vi "DCM Constants and GUIDs.vi"() -> ()   [LabVIEW 2016, in "DCM Shared.lvlib"]
uses:
  DCM Shared.lvlib
  Types/Channel.ctl
panel:
  in  "Tab Control":T1(tab)
  in  "GUID.Aux":string="4ae80cd4-ec55-4ec1-b4bb-2001c61b6b14"
  in  "GUID.EnableDisableKnock":string="8a875cae-6cab-46b6-b4a7-b8cdf862ac1d"
  in  "GUID.Knock Disabled":string="a0532e73-7f55-4d0e-9b0f-dca8ef6be3da"
  in  "GUID.EnableDisableSkipfire":string="bbdda3d2-34c9-4362-989f-a288134847eb"
  in  "GUID.Skipfire Disabled":string="c54507d4-3cef-40f9-a6c1-87c28a1ea6a0"
  in  "GUID.Skipfire":string="1ac39163-a8a7-406d-af0d-2094f9d35b5e"
  in  "GUID.HH Scope":string="6092b7fa-6603-4513-a21d-943bed09a899"
  in  "GUID.EnableDisableESTTL":string="e242de91-e1a9-42ca-a209-c7115f438d37"
  in  "GUID.ESTTL Disabled":string="2ad3d1d5-7c00-47db-b770-0db9f08c91b8"
  in  "GUID.EnableDisableDiffIO":string="917ddf8a-c153-44a1-b2f2-6ada7a308212"
  in  "GUID.Differential IO Disabled":string="faee9789-46db-458a-959a-05641d5004e2"
  in  "GUID.EnableDisableHalfH":string="e0f39d5d-4753-4142-ac63-84ba8dc69499"
  in  "GUID.Half-H Disabled":string="e47a1de0-27ee-4cc7-82d3-285b476618bb"
  in  "GUID.EnableDisableBankB":string="4d434972-4aa6-45af-92be-8034ae6f2b6c"
  in  "GUID.EnableDisableBankA":string="46df0418-deb6-4d59-8d20-0ae52d1e3a0a"
  in  "GUID.DI (Bank B) Disabled":string="ba7b8b99-1cfb-447e-88fa-e4ec3244df79"
  in  "GUID.DI (Bank A) Disabled":string="0515dfd1-3106-4f60-bfdc-e9560b274cce"
  in  "GUID.Knock":string="19fe4c45-3921-4e09-b642-633bf2891a16"
  in  "GUID.UEGO":string="5fb3e6f2-894a-4878-a5bb-3886d90bfc3e"
  in  "GUID.VR-Hall":string="cf54691f-9754-47a4-ae55-d66845591b75"
  in  "GUID.ESTTL":string="38e1f48f-5a27-4a02-97fd-d113d0b0a1a5"
  in  "GUID.Wvfrm Del Prot":string="7d419a3c-75c3-4347-a0a2-a7591295b469"
  in  "GUID.System":string="d2cc065c-850f-4944-a4c9-610c3de05f2d"
  in  "GUID.Sect Write Del Prot":string="e1e0ebe0-7744-485e-8dcf-da45db37f6d7"
  in  "GUID.DI Scope":string="4a79ddeb-a706-489a-9bbf-290de6baccd6"
  in  "GUID.EnableDisableMain":string="f10bd84a-c71b-4bab-a7fa-9098b9fd69a6"
  in  "GUID.Status":string="39854a26-935c-4763-8ef8-825ef45b52f8"
  in  "GUID.Main Disabled":string="f599dfb9-ed26-42aa-8cdc-f57f090e1b11"
  in  "GUID.Differential IO":string="2628923f-4c3d-4e64-9018-fe4e0bf24e80"
  in  "GUID.Half-H":string="f16175a1-fad9-427d-a4ec-263940a8031d"
  in  "GUID.DI (Bank B)":string="a63b3095-c73b-454f-88f9-68383dab1f80"
  in  "GUID.DI (Bank A)":string="f8d973f8-2e11-4124-aa70-a6fee72385c1"
  in  "GUID.EPTx":string="a5efee57-fd86-4078-b618-b0705acc47b3"
  in  "GUID.Sect Read Del Prot":string="6b94385d-a8fe-4299-8780-02040b069697"
  in  "GUID.Chan Del Prot":string="c457cef7-60a4-4609-953f-49bd172293ff"
  in  "GUID.Main Enabled":string="1e4c05d8-9abf-4fec-b650-9db71821173c"
  in  "Constant.Aux Inputs":string="Aux Inputs"
  in  "Constant.Skip Fire":string="Skip Fire"
  in  "Constant.Select 2":string="Select"
  in  "Constant.Filters":string="Filters"
  in  "Constant.Half-H Scope":string="Half-H Scope"
  in  "Constant.Command DI":string="Command DI"
  in  "Constant.Command Pump":string="Command Pump"
  in  "Constant.Knock Intensity":string="Knock Intensity"
  in  "Constant.Knock":string="Knock"
  in  "Constant.Diagnostics":string="Diagnostics"
  in  "Constant.Temperature":string="Temperature"
  in  "Constant.ESTTL":string="ESTTL"
  in  "Constant.VR-Hall":string="VR-Hall"
  in  "Constant.UEGO":string="UEGO"
  in  "Constant.Invalid Selection":string="Invalid Selection"
  in  "Constant.WrongMode":string="Selected Configuration invalid for Sync Pump operation."
  in  "Constant.Select":string="Select"
  in  "Constant.User OS":string="User OS"
  in  "Constant.Config":string="Config"
  in  "Constant.DisableChannels":string="Disabling channels will delete all relevant configuration information. Proceed?"
  in  "Constant.Input State":string="Input State"
  in  "Constant.Clear Faults":string="Clear Faults"
  in  "Constant.Debug":string="Debug"
  in  "Constant.Mux ADC":string="Mux ADC"
  in  "Constant.System":string="System"
  in  "Constant.DI Scope":string="DI Scope"
  in  "Constant.Description":string="Description"
  in  "Constant.HH Command":string="HH Command"
  in  "Constant.Results":string="Results"
  in  "Constant.Setup":string="Setup"
  in  "Constant.Command":string="Command"
  in  "Constant.EPTx":string="EPTx"
  in  "Constant.invalid bitfile":string="Invalid Bitfile"
  in  "Constant.ConfirmDelete":string="Confirm delete configuration"
  in  "Constant.ChangeBitfile":string="Changing bitfile will delete all relevant configuration information. Proceed?"
  in  "Constant.RemoveBitfile":string="Removing the bitfile path will delete all configuration information. Proceed?"
  in  "Constant.Status":string="Status"
  in  "Constant.Waveforms":string="Waveforms"
  in  "Constant.Thresholding":string="Thresholding"
  in  "Constant.Differential IO":string="Differential I/O"
  in  "Constant.Half-H":string="Half-H"
  in  "Constant.DI (Bank B)":string="DI (Bank B)"
  in  "Constant.DI (Bank A)":string="DI (Bank A)"
  in  "Constant.Data":string="Data"
  in  "Constant.Control":string="Control"
  in  "Constant.not present":string="- not added -"
  in  "ChanList.DI Status":T2[](array[typedef])=[{"Name"="A Run State", "Units"="enum", "Default"=0.0, "Description"="Indicates DI Bank A run status. [Idle|Warmup|Ready to Inject|Cooldown]"}, {"Name"="B Run State", "Units"="enum", "Default"=0.0, "Description"="Indicates DI Bank B run status. [Idle|Warmup|Ready to Inject|Cooldown]"}]
  in  "ChanList.Knock Controls":T2[](array[typedef])=[{"Name"="Low Cutoff", "Units"="Hz", "Default"=4000.0, "Description"="Sets the low cutoff frequency for knock calculations."}, {"Name"="High Cutoff", "Units"="Hz", "Default"=10000.0, "Description"="Sets the high cutoff frequency for knock calculations."}, {"Name"="Threshold", "Units"="", "Default"=1.0, "Description"="Sets the minimum calculation result which represents a knocking condition."}, {"Name"="Knock Start", "Units"="CAD", "Default"=0.0, "Description"="Sets the start of the knock sampling window."}, {"Name"="Knock End", "Units"="CAD", "Default"=0.0, "Description"="Sets the end of the knock sampling window."}, {"Name"="Reference Start", "Units"="CAD", "Default"=0.0, "Description"="Sets the start of the reference sampling window."}, {"Name"="Reference End", "Units"="CAD", "Default"=0.0, "Description"="Sets the end of the reference sampling window."}]
  in  "ChanList.HH Scope":T2[](array[typedef])=[{"Name"="Capture Enable", "Units"="bool", "Default"=0.0, "Description"="Enables HH-ADC Scope capture."}, {"Name"="Capture Event", "Units"="enum", "Default"=0.0, "Description"="Selects the HH-ADC scope trigger event."}, {"Name"="Capture Length", "Units"="s", "Default"=0.0, "Description"="Sets the length of the HH Scope waveform buffer."}, {"Name"="dt", "Units"="s", "Default"=2e-07, "Description"="Indicates the HH Scope dt in seconds."}]
  in  "ChanList.Knock Intensity":T2[](array[typedef])=[{"Name"="Knock Intensity 1", "Units"="", "Default"=0.0, "Description"="Indicates the intensity of knock reported by the FPGA."}, {"Name"="Knock Intensity 2", "Units"="", "Default"=0.0, "Description"="Indicates the intensity of knock reported by the FPGA."}, {"Name"="Knock Intensity 3", "Units"="", "Default"=0.0, "Description"="Indicates the intensity of knock reported by the FPGA."}, {"Name"="Knock Intensity 4", "Units"="", "Default"=0.0, "Description"="Indicates the intensity of knock reported by the FPGA."}, {"Name"="Knock Intensity 5", "Units"="", "Default"=0.0, "Description"="Indicates the intensity of knock reported by the FPGA."}, {"Name"="Knock Intensity 6", "Units"="", "Default"=0.0, "Description"="Indicates the intensity of knock reported by the FPGA."}, {"Name"="Knock Intensity 7", "Units"="", "Default"=0.0, "Description"="Indicates the intensity of knock reported by the FPGA."}, {"Name"="Knock Intensity 8", "Units"="", "Default"=0.0, "Description"="Indicates the intensity of knock reported by the FPGA."}, {"Name"="Knock Intensity 9", "Units"="", "Default"=0.0, "Description"="Indicates the intensity of knock reported by the FPGA."}, {"Name"="Knock Intensity 10", "Units"="", "Default"=0.0, "Description"="Indicates the intensity of knock reported by the FPGA."}, {"Name"="Knock Intensity 11", "Units"="", "Default"=0.0, "Description"="Indicates the intensity of knock reported by the FPGA."}, {"Name"="Knock Intensity 12", "Units"="", "Default"=0.0, "Description"="Indicates the intensity of knock reported by the FPGA."}, {"Name"="Knock Intensity 13", "Units"="", "Default"=0.0, "Description"="Indicates the intensity of knock reported by the FPGA."}, {"Name"="Knock Intensity 14", "Units"="", "Default"=0.0, "Description"="Indicates the intensity of knock reported by the FPGA."}, {"Name"="Knock Intensity 15", "Units"="", "Default"=0.0, "Description"="Indicates the intensity of knock reported by the FPGA."}, {"Name"="Knock Intensity 16", "Units"="", "Default"=0.0, "Description"="Indicates the intensity of knock reported by the FPGA."}]
  in  "ChanList.Knock Result":T2[](array[typedef])=[{"Name"="Knock 1", "Units"="bool", "Default"=0.0, "Description"="Indicates the presence of knock above the calibrated threshold."}, {"Name"="Knock 2", "Units"="bool", "Default"=0.0, "Description"="Indicates the presence of knock above the calibrated threshold."}, {"Name"="Knock 3", "Units"="bool", "Default"=0.0, "Description"="Indicates the presence of knock above the calibrated threshold."}, {"Name"="Knock 4", "Units"="bool", "Default"=0.0, "Description"="Indicates the presence of knock above the calibrated threshold."}, {"Name"="Knock 5", "Units"="bool", "Default"=0.0, "Description"="Indicates the presence of knock above the calibrated threshold."}, {"Name"="Knock 6", "Units"="bool", "Default"=0.0, "Description"="Indicates the presence of knock above the calibrated threshold."}, {"Name"="Knock 7", "Units"="bool", "Default"=0.0, "Description"="Indicates the presence of knock above the calibrated threshold."}, {"Name"="Knock 8", "Units"="bool", "Default"=0.0, "Description"="Indicates the presence of knock above the calibrated threshold."}, {"Name"="Knock 9", "Units"="bool", "Default"=0.0, "Description"="Indicates the presence of knock above the calibrated threshold."}, {"Name"="Knock 10", "Units"="bool", "Default"=0.0, "Description"="Indicates the presence of knock above the calibrated threshold."}, {"Name"="Knock 11", "Units"="bool", "Default"=0.0, "Description"="Indicates the presence of knock above the calibrated threshold."}, {"Name"="Knock 12", "Units"="bool", "Default"=0.0, "Description"="Indicates the presence of knock above the calibrated threshold."}, {"Name"="Knock 13", "Units"="bool", "Default"=0.0, "Description"="Indicates the presence of knock above the calibrated threshold."}, {"Name"="Knock 14", "Units"="bool", "Default"=0.0, "Description"="Indicates the presence of knock above the calibrated threshold."}, {"Name"="Knock 15", "Units"="bool", "Default"=0.0, "Description"="Indicates the presence of knock above the calibrated threshold."}, {"Name"="Knock 16", "Units"="bool", "Default"=0.0, "Description"="Indicates the presence of knock above the calibrated threshold."}]
  in  "ChanList.VR-Hall":T2[](array[typedef])=[{"Name"="Clear Faults", "Units"="bool", "Default"=0.0, "Description"="Clears a fault condition where an input voltage is too negative to safely engage pull-up resistor on the positive(+) side of input channels."}]
  in  "ChanList.UEGO Temp":T2[](array[typedef])=[{"Name"="UEGO1Temp", "Units"="C", "Default"=0.0, "Description"="The controlled temperature, in degrees Celsius, of the wide-band sensor element.\n \nFor LSU 4.2 sensors the temperature setpoint is 750 degrees C.\n \nFor LSU 4.9 sensors the temperature setpoint is 780 degrees C.\n \nThe allowable voltage range for LSU 4.X sensor heater operation is 8.0-16.5V, even though the O2 Sensor Module will operate from 7-32V supply.  If the module supply voltage exceeds 16.5V, the sensor heater will be disabled."}, {"Name"="UEGO2Temp", "Units"="C", "Default"=0.0, "Description"="The controlled temperature, in degrees Celsius, of the wide-band sensor element.\n \nFor LSU 4.2 sensors the temperature setpoint is 750 degrees C.\n \nFor LSU 4.9 sensors the temperature setpoint is 780 degrees C.\n \nThe allowable voltage range for LSU 4.X sensor heater operation is 8.0-16.5V, even though the O2 Sensor Module will operate from 7-32V supply.  If the module supply voltage exceeds 16.5V, the sensor heater will be disabled."}, {"Name"="UEGO1Hot", "Units"="bool", "Default"=0.0, "Description"="Indicates whether the sensor ceramic temperature has reached the target after enabled.  Lambda results are valid when UEGOXHot is TRUE.\n \nFor LSU 4.2 :\nA temperature change of the sensor ceramic gives a deviation of the sensor output signal of approximately 6%/100C.\nTarget ceramic temperature: 750C\nUEGOHot transitions from FALSE to TRUE when the temperature reaches the target temperature for the first time after enabled.\nUEGOHot transitions from TRUE to FALSE when the sensor or module are disabled, or the battery voltage is measured out of range.\n \nFor LSU 4.9 :\nA temperature change of the sensor ceramic gives a deviation of the sensor output signal of approximately 4%/100C.\nTarget ceramic temperature: 780C\nUEGOHot transitions from FALSE to TRUE when the temperature reaches the target temperature for the first time after enabled.\nUEGOHot transitions from TRUE to FALSE when the sensor or module are disabled, or the battery voltage is measured out of range.\n \nThe allowable voltage range for LSU 4.X sensor heater operation is 8.0-16.5V, even though the O2 Sensor Module will operate from 7-32V supply.  If the module supply voltage exceeds 16.5V, the sensor heater will be disabled."}, {"Name"="UEGO2Hot", "Units"="bool", "Default"=0.0, "Description"="Indicates whether the sensor ceramic temperature has reached the target after enabled.  Lambda results are valid when UEGOXHot is TRUE.\n \nFor LSU 4.2 :\nA temperature change of the sensor ceramic gives a deviation of the sensor output signal of approximately 6%/100C.\nTarget ceramic temperature: 750C\nUEGOHot transitions from FALSE to TRUE when the temperature reaches the target temperature for the first time after enabled.\nUEGOHot transitions from TRUE to FALSE when the sensor or module are disabled, or the battery voltage is measured out of range.\n \nFor LSU 4.9 :\nA temperature change of the sensor ceramic gives a deviation of the sensor output signal of approximately 4%/100C.\nTarget ceramic temperature: 780C\nUEGOHot transitions from FALSE to TRUE when the temperature reaches the target temperature for the first time after enabled.\nUEGOHot transitions from TRUE to FALSE when the sensor or module are disabled, or the battery voltage is measured out of range.\n \nThe allowable voltage range for LSU 4.X sensor heater operation is 8.0-16.5V, even though the O2 Sensor Module will operate from 7-32V supply.  If the module supply voltage exceeds 16.5V, the sensor heater will be disabled."}]
  in  "ChanList.UEGO Diagnostics":T2[](array[typedef])=[{"Name"="UEGO1SensorFault", "Units"="enum", "Default"=0.0, "Description"="NO FAULT: No faults exist with the sensor signal wires. \n \nSHORT TO GND OR BATT: A short to ground or battery is present on one of the sensor signal wires."}, {"Name"="UEGO2SensorFault", "Units"="enum", "Default"=0.0, "Description"="NO FAULT: No faults exist with the sensor signal wires. \n \nSHORT TO GND OR BATT: A short to ground or battery is present on one of the sensor signal wires."}, {"Name"="UEGO1HeaterFault", "Units"="enum", "Default"=0.0, "Description"="NO FAULT: No faults exist with the sensor heater wires. \n \nSHORT TO GROUND: A short to ground is present on one of the sensor heater wires. \n \nOPEN CIRCUIT: An open circuit is present on one of the sensor heater wires. \n \nSHORT TO BATTERY: A short to battery is present on one of the sensor heater wires."}, {"Name"="UEGO2HeaterFault", "Units"="enum", "Default"=0.0, "Description"="NO FAULT: No faults exist with the sensor heater wires. \n \nSHORT TO GROUND: A short to ground is present on one of the sensor heater wires. \n \nOPEN CIRCUIT: An open circuit is present on one of the sensor heater wires. \n \nSHORT TO BATTERY: A short to battery is present on one of the sensor heater wires."}, {"Name"="UEGOFuseStatus", "Units"="enum", "Default"=0.0, "Description"="A single fuse is located in the module circuit which feeds battery voltage to both sensor heaters. \n \nFUSE OK: The heater circuit fuse is OK. \n \nFUSE BLOWN: The heater circuit fuse is blown."}, {"Name"="Battery", "Units"="V", "Default"=0.0, "Description"="Battery voltage sensed internal to the module while enabled."}, {"Name"="LSUType", "Units"="enum", "Default"=0.0, "Description"="Indicates the UEGO sensor type supported by the module according to an internal mechanical switch.\n \nFALSE (default switch position): Module switch is configured for the Bosch LSU 4.9 sensor.\n \nTRUE: Module switch is configured for the Bosch LSU 4.2 sensor.\n \nNote: The module can only support one UEGO sensor type.  It is not possible to configure the two UEGO sensor channels for different sensor types.\n \nNote: The NI 9757 module has a single internal mechanical switch that determines the supported sensor type by selecting the correct passive components for the sensors.  This switch is configured from the factory to support the Bosch LSU 4.9 sensor. The UEGO Diagnostics cluster reports the switch configuration.\n \nWARNING: The module does not automatically detect the type of UEGO sensor wired to the module.  If the connected sensor type does not match the module mechanical switch setting, damage may occur to the sensor.  In particular, an LSU 4.9 sensor operated while the switch is set to LSU 4.2 will cause the 4.9 sensor to overheat."}]
  in  "ChanList.UEGO Results":T2[](array[typedef])=[{"Name"="UEGO1Lambda", "Units"="", "Default"=0.0, "Description"="The actual air-fuel mass ratio divided by the stoichiometric air-fuel mass ratio. Lambda is equivalent to 1/Phi."}, {"Name"="UEGO1Phi", "Units"="", "Default"=0.0, "Description"="The actual fuel/air mass ratio divided by the stoichiometric fuel-air mass ratio. Phi is equivalent to 1/Lambda."}, {"Name"="UEGO1AFRatio", "Units"="", "Default"=0.0, "Description"="The actual air-fuel mass ratio."}, {"Name"="UEGO1Ip", "Units"="mA", "Default"=0.0, "Description"="The pump current required for maintaining a reference voltage of 450 millivolts across the wide-band sensor element. This is also the current required for maintaining a stoichiometric gas mixture within the sensor element."}, {"Name"="UEGO2Lambda", "Units"="", "Default"=0.0, "Description"="The actual air-fuel mass ratio divided by the stoichiometric air-fuel mass ratio. Lambda is equivalent to 1/Phi."}, {"Name"="UEGO2Phi", "Units"="", "Default"=0.0, "Description"="The actual fuel/air mass ratio divided by the stoichiometric fuel-air mass ratio. Phi is equivalent to 1/Lambda."}, {"Name"="UEGO2AFRatio", "Units"="", "Default"=0.0, "Description"="The actual air-fuel mass ratio."}, {"Name"="UEGO2Ip", "Units"="mA", "Default"=0.0, "Description"="The pump current required for maintaining a reference voltage of 450 millivolts across the wide-band sensor element. This is also the current required for maintaining a stoichiometric gas mixture within the sensor element."}]
  in  "ChanList.UEGO Control":T2[](array[typedef])=[{"Name"="UEGO1Enable", "Units"="bool", "Default"=0.0, "Description"="Enables UEGO1 sensor"}, {"Name"="UEGO2Enable", "Units"="bool", "Default"=0.0, "Description"="Enables UEGO2 sensor"}, {"Name"="UEGO1Range", "Units"="bool", "Default"=0.0, "Description"="Adjusts the amplifaction range for lambda measurement.  Two amplification modes are available:  One mode, having an amplifier gain factor of 8, allows for measurements of lambda from 0.65 to air.  The other mode, having an amplifier gain factor of 17, allows for measurements of lambda = 0.75 to air.  It is recommended to use the gain factor of 17 for operation above lambda = 1.5.  This gain factor provides better resolution in the lean region.  The gain factor can be changed at any time during operation.\n \nFALSE (Gain factor = 8): Allows measurement of lambda from 0.65 to air.\n \nTRUE (Gain factor = 17): Allows measurement of lambda from 0.75 to air."}, {"Name"="UEGO2Range", "Units"="bool", "Default"=0.0, "Description"="Adjusts the amplifaction range for lambda measurement.  Two amplification modes are available:  One mode, having an amplifier gain factor of 8, allows for measurements of lambda from 0.65 to air.  The other mode, having an amplifier gain factor of 17, allows for measurements of lambda = 0.75 to air.  It is recommended to use the gain factor of 17 for operation above lambda = 1.5.  This gain factor provides better resolution in the lean region.  The gain factor can be changed at any time during operation.\n \nFALSE (Gain factor = 8): Allows measurement of lambda from 0.65 to air.\n \nTRUE (Gain factor = 17): Allows measurement of lambda from 0.75 to air."}, {"Name"="Filter Cutoff", "Units"="Hz", "Default"=10.0, "Description"="Second-order Butterworth lowpass filter cutoff frequency which applies to all UEGO signals."}]
  in  "ChanList.UserOS":T2[](array[typedef])=[{"Name"="User OS", "Units"="bool", "Default"=0.0, "Description"="Triggers a one-shot injection on OS-enabled channels on rising edge."}, {"Name"="User OS Time", "Units"="s", "Default"=0.0, "Description"="One-shot duration in seconds."}]
  in  "ChanList.HH Status":T2[](array[typedef])=[{"Name"="Current", "Units"="A", "Default"=0.0, "Description"="Instantaneous channel current in amps."}, {"Name"="Config Error", "Units"="bool", "Default"=0.0, "Description"="Indicates a configuration error on this channel."}, {"Name"="Short Fault", "Units"="bool", "Default"=0.0, "Description"="Indicates a short is detected on this channel."}, {"Name"="Open Fault", "Units"="bool", "Default"=0.0, "Description"="Indicates an open circuit was detected on this channel."}, {"Name"="Period Min", "Units"="A", "Default"=0.0, "Description"="Min current measured during one command period."}, {"Name"="Period Max", "Units"="A", "Default"=0.0, "Description"="Max current measured during one command period."}, {"Name"="Period Avg", "Units"="A", "Default"=0.0, "Description"="Average current mesasured during one command period"}, {"Name"="On Avg", "Units"="A", "Default"=0.0, "Description"="Average current measured during the on portion of one command period."}]
  in  "ChanList.DiffIO In":T2[](array[typedef])=[{"Name"="DI 1", "Units"="bool", "Default"=0.0, "Description"="Digital state of Diff IO channel input."}, {"Name"="DI 2", "Units"="bool", "Default"=0.0, "Description"="Digital state of Diff IO channel input."}, {"Name"="DI 3", "Units"="bool", "Default"=0.0, "Description"="Digital state of Diff IO channel input."}, {"Name"="DI 4", "Units"="bool", "Default"=0.0, "Description"="Digital state of Diff IO channel input."}, {"Name"="DI 5", "Units"="bool", "Default"=0.0, "Description"="Digital state of Diff IO channel input."}, {"Name"="DI 6", "Units"="bool", "Default"=0.0, "Description"="Digital state of Diff IO channel input."}, {"Name"="DI 7", "Units"="bool", "Default"=0.0, "Description"="Digital state of Diff IO channel input."}, {"Name"="DI 8", "Units"="bool", "Default"=0.0, "Description"="Digital state of Diff IO channel input."}]
  in  "ChanList.DI Fault Clear":T2[](array[typedef])=[{"Name"="Channel 1", "Units"="bool", "Default"=0.0, "Description"="Clears DI faults on this channel."}, {"Name"="Channel 2", "Units"="bool", "Default"=0.0, "Description"="Clears DI faults on this channel."}, {"Name"="Channel 3", "Units"="bool", "Default"=0.0, "Description"="Clears DI faults on this channel."}, {"Name"="Channel 4", "Units"="bool", "Default"=0.0, "Description"="Clears DI faults on this channel."}, {"Name"="Channel 5", "Units"="bool", "Default"=0.0, "Description"="Clears DI faults on this channel."}, {"Name"="Channel 6", "Units"="bool", "Default"=0.0, "Description"="Clears DI faults on this channel."}, {"Name"="Channel 7", "Units"="bool", "Default"=0.0, "Description"="Clears DI faults on this channel."}, {"Name"="Channel 8", "Units"="bool", "Default"=0.0, "Description"="Clears DI faults on this channel."}]
  in  "ChanList.DI Config":T2[](array[typedef])=[{"Name"="Power Supply Enable", "Units"="bool", "Default"=0.0, "Description"="Enables high voltage power supply (0=F, 1=T)."}, {"Name"="Injection Enable", "Units"="bool", "Default"=0.0, "Description"="Enables injection (0=F, 1=T)."}, {"Name"="High Voltage Target", "Units"="V", "Default"=75.0, "Description"="Sets the high voltage power supply target in volts."}]
  in  "ChanList.DI Scope":T2[](array[typedef])=[{"Name"="Capture Enable", "Units"="bool", "Default"=0.0, "Description"="Enables DI-ADC Scope capture."}, {"Name"="Capture Event", "Units"="enum", "Default"=0.0, "Description"="Selects the DI-ADC scope trigger event."}, {"Name"="Capture Length", "Units"="s", "Default"=0.0, "Description"="Sets the length of the DI Scope waveform buffer."}, {"Name"="Channel 1", "Units"="enum", "Default"=0.0, "Description"="Selects the desired channel for the high-speed DI ADC.\n\n0: Lowside Current A1\n1: Lowside Current A2\n2: Lowside Current A3\n3: Lowside Current A4\n4: Lowside Current A5\nA: Piezo Voltage A1\nB: Piezo Voltage A2\nC: Piezo Voltage A3\nD: Piezo Voltage A4\n6: Solenoid Voltage A1\n7: Solenoid Voltage A2\n8: Solenoid Voltage A3\n9: Solenoid Voltage A4\n60: High Voltage A1\n70: High Voltage A2\nE: High Voltage A\n-----------------------------\n13: Lowside Current B1\n12: Lowside Current B2\n11: Lowside Current B3\n10: Lowside Current B4\n14: Lowside Current B5\n19: Piezo Voltage B1\n18: Piezo Voltage B2\n17: Piezo Voltage B3\n16: Piezo Voltage B4\n1F: Solenoid Voltage B1\n1E: Solenoid Voltage B2\n1D: Solenoid Voltage B3\n1C: Solenoid Voltage B4\n90: High Voltage B1\n80: High Voltage B2\nF: High Voltage B\n-----------------------------\n1A: Analog Input 1\n1B: Analog Input 2\nA0: Drive Power"}, {"Name"="Channel 2", "Units"="enum", "Default"=0.0, "Description"="Selects the desired channel for the high-speed DI ADC.\n\n0: Lowside Current A1\n1: Lowside Current A2\n2: Lowside Current A3\n3: Lowside Current A4\n4: Lowside Current A5\nA: Piezo Voltage A1\nB: Piezo Voltage A2\nC: Piezo Voltage A3\nD: Piezo Voltage A4\n6: Solenoid Voltage A1\n7: Solenoid Voltage A2\n8: Solenoid Voltage A3\n9: Solenoid Voltage A4\n60: High Voltage A1\n70: High Voltage A2\nE: High Voltage A\n-----------------------------\n13: Lowside Current B1\n12: Lowside Current B2\n11: Lowside Current B3\n10: Lowside Current B4\n14: Lowside Current B5\n19: Piezo Voltage B1\n18: Piezo Voltage B2\n17: Piezo Voltage B3\n16: Piezo Voltage B4\n1F: Solenoid Voltage B1\n1E: Solenoid Voltage B2\n1D: Solenoid Voltage B3\n1C: Solenoid Voltage B4\n90: High Voltage B1\n80: High Voltage B2\nF: High Voltage B\n-----------------------------\n1A: Analog Input 1\n1B: Analog Input 2\nA0: Drive Power"}, {"Name"="Channel 3", "Units"="enum", "Default"=0.0, "Description"="Selects the desired channel for the high-speed DI ADC.\n\n0: Lowside Current A1\n1: Lowside Current A2\n2: Lowside Current A3\n3: Lowside Current A4\n4: Lowside Current A5\nA: Piezo Voltage A1\nB: Piezo Voltage A2\nC: Piezo Voltage A3\nD: Piezo Voltage A4\n6: Solenoid Voltage A1\n7: Solenoid Voltage A2\n8: Solenoid Voltage A3\n9: Solenoid Voltage A4\n60: High Voltage A1\n70: High Voltage A2\nE: High Voltage A\n-----------------------------\n13: Lowside Current B1\n12: Lowside Current B2\n11: Lowside Current B3\n10: Lowside Current B4\n14: Lowside Current B5\n19: Piezo Voltage B1\n18: Piezo Voltage B2\n17: Piezo Voltage B3\n16: Piezo Voltage B4\n1F: Solenoid Voltage B1\n1E: Solenoid Voltage B2\n1D: Solenoid Voltage B3\n1C: Solenoid Voltage B4\n90: High Voltage B1\n80: High Voltage B2\nF: High Voltage B\n-----------------------------\n1A: Analog Input 1\n1B: Analog Input 2\nA0: Drive Power"}, {"Name"="Channel 4", "Units"="enum", "Default"=0.0, "Description"="Selects the desired channel for the high-speed DI ADC.\n\n0: Lowside Current A1\n1: Lowside Current A2\n2: Lowside Current A3\n3: Lowside Current A4\n4: Lowside Current A5\nA: Piezo Voltage A1\nB: Piezo Voltage A2\nC: Piezo Voltage A3\nD: Piezo Voltage A4\n6: Solenoid Voltage A1\n7: Solenoid Voltage A2\n8: Solenoid Voltage A3\n9: Solenoid Voltage A4\n60: High Voltage A1\n70: High Voltage A2\nE: High Voltage A\n-----------------------------\n13: Lowside Current B1\n12: Lowside Current B2\n11: Lowside Current B3\n10: Lowside Current B4\n14: Lowside Current B5\n19: Piezo Voltage B1\n18: Piezo Voltage B2\n17: Piezo Voltage B3\n16: Piezo Voltage B4\n1F: Solenoid Voltage B1\n1E: Solenoid Voltage B2\n1D: Solenoid Voltage B3\n1C: Solenoid Voltage B4\n90: High Voltage B1\n80: High Voltage B2\nF: High Voltage B\n-----------------------------\n1A: Analog Input 1\n1B: Analog Input 2\nA0: Drive Power"}, {"Name"="dt", "Units"="s", "Default"=2e-07, "Description"="Indicates the DI Scope dt in seconds."}]
  in  "ChanList.System Control":T2[](array[typedef])=[{"Name"="MPRD", "Units"="bool", "Default"=0.0, "Description"="Main Power Relay (0=F, 1=T)."}, {"Name"="User LED 1", "Units"="enum", "Default"=0.0, "Description"="0=Off, 1=Yellow, 2=Green"}, {"Name"="User LED 2", "Units"="enum", "Default"=0.0, "Description"="0=Off, 1=Yellow, 2=Green"}]
  in  "ChanList.Status Chans":T2[](array[typedef])=[{"Name"="Cmd - Status code", "Units"="", "Default"=0.0, "Description"="Status code of the custom device. A negative value indicates failure. A positive value indicates warning."}, {"Name"="Cmd - Loop duration", "Units"="ns", "Default"=0.0, "Description"="Duration of the custom device loop in nanoseconds. This can be monitored to measure performance relative to the desired loop rate."}, {"Name"="Cmd - Late count", "Units"="", "Default"=0.0, "Description"="Number of times the custom device loop has gone late."}, {"Name"="Sys - Status code", "Units"="", "Default"=0.0, "Description"="Status code of the custom device. A negative value indicates failure. A positive value indicates warning."}, {"Name"="Sys - Loop duration", "Units"="ns", "Default"=0.0, "Description"="Duration of the custom device loop in nanoseconds. This can be monitored to measure performance relative to the desired loop rate."}, {"Name"="Sys - Late count", "Units"="", "Default"=0.0, "Description"="Number of times the custom device loop has gone late."}]
  in  "ChanList.EPTx Data":T2[](array[typedef])=[{"Name"="Sync", "Units"="bool", "Default"=0.0, "Description"="Indicates that EPTx is synced."}, {"Name"="CurrentCAD", "Units"="CAD", "Default"=0.0, "Description"="Current engine position in CAD."}, {"Name"="Speed", "Units"="RPM", "Default"=0.0, "Description"="Reported engine speed from EPTx."}, {"Name"="Config", "Units"="bool", "Default"=0.0, "Description"="Indicates EPTx is being configured."}, {"Name"="Rcvg Primary", "Units"="bool", "Default"=0.0, "Description"="Indicates that EPTx is seeing an incoming primary signal."}, {"Name"="Stall", "Units"="bool", "Default"=0.0, "Description"="Indicates the reported speed has fallen below the EPTx stall speed."}, {"Name"="Overflow Error", "Units"="bool", "Default"=0.0, "Description"="Indicates an Overflow Error on the EPTx FPGA core."}, {"Name"="Ratio Error", "Units"="bool", "Default"=0.0, "Description"="Indicates EPTx measured an unexpected signal event ratio."}, {"Name"="Pattern Error", "Units"="bool", "Default"=0.0, "Description"="Indicates EPTx measured a signal event ratio outside of the expected SER pattern."}, {"Name"="Aux Warning", "Units"="bool", "Default"=0.0, "Description"="Indicates an Aux signal was measured outside of expected bounds after sync."}, {"Name"="Watchdog Error", "Units"="bool", "Default"=0.0, "Description"="Indicates the RT watchdog has not been received by the FPGA target."}, {"Name"="Loading", "Units"="bool", "Default"=0.0, "Description"="Indicates the EPTx RT core is loading EPTx configuration data to the FPGA."}]
  in  "ChanList.EPTx Controls":T2[](array[typedef])=[{"Name"="Reload EPTx", "Units"="bool", "Default"=0.0, "Description"="Reloads EPTx Configuration"}, {"Name"="Sync Enable", "Units"="bool", "Default"=0.0, "Description"="Enables EPTx Sync."}, {"Name"="Clear Errors", "Units"="bool", "Default"=0.0, "Description"="Clears EPTx error on RT and FPGA."}, {"Name"="Sim Enable", "Units"="bool", "Default"=0.0, "Description"="Enables internal EPTx simulation of engine speed."}, {"Name"="Sim Speed", "Units"="RPM", "Default"=1000.0, "Description"="Desired simulated speed."}]
  in  "WvfrmList.HH Scope":T2[](array[typedef])=[{"Name"="Channel 1", "Units"="V", "Default"=0.0, "Description"="Channel 1 Data"}, {"Name"="Channel 2", "Units"="V", "Default"=0.0, "Description"="Channel 2 Data"}, {"Name"="Channel 3", "Units"="V", "Default"=0.0, "Description"="Channel 3 Data"}, {"Name"="Channel 4", "Units"="V", "Default"=0.0, "Description"="Channel 4 Data"}, {"Name"="Channel 5", "Units"="V", "Default"=0.0, "Description"="Channel 5 Data"}, {"Name"="Channel 6", "Units"="V", "Default"=0.0, "Description"="Channel 6 Data"}, {"Name"="Channel 7", "Units"="V", "Default"=0.0, "Description"="Channel 7Data"}, {"Name"="Channel 8", "Units"="V", "Default"=0.0, "Description"="Channel 8 Data"}, {"Name"="Channel 9", "Units"="V", "Default"=0.0, "Description"="Channel 9 Data"}, {"Name"="Channel 10", "Units"="V", "Default"=0.0, "Description"="Channel 10 Data"}, {"Name"="Channel 11", "Units"="V", "Default"=0.0, "Description"="Channel 11 Data"}, {"Name"="Channel 12", "Units"="V", "Default"=0.0, "Description"="Channel 12 Data"}]
  in  "WvfrmList.DI Scope":T2[](array[typedef])=[{"Name"="Channel 1", "Units"="V", "Default"=0.0, "Description"="Channel 1 Data"}, {"Name"="Channel 2", "Units"="V", "Default"=0.0, "Description"="Channel 2 Data"}, {"Name"="Channel 3", "Units"="V", "Default"=0.0, "Description"="Channel 3 Data"}, {"Name"="Channel 4", "Units"="V", "Default"=0.0, "Description"="Channel 4 Data"}]
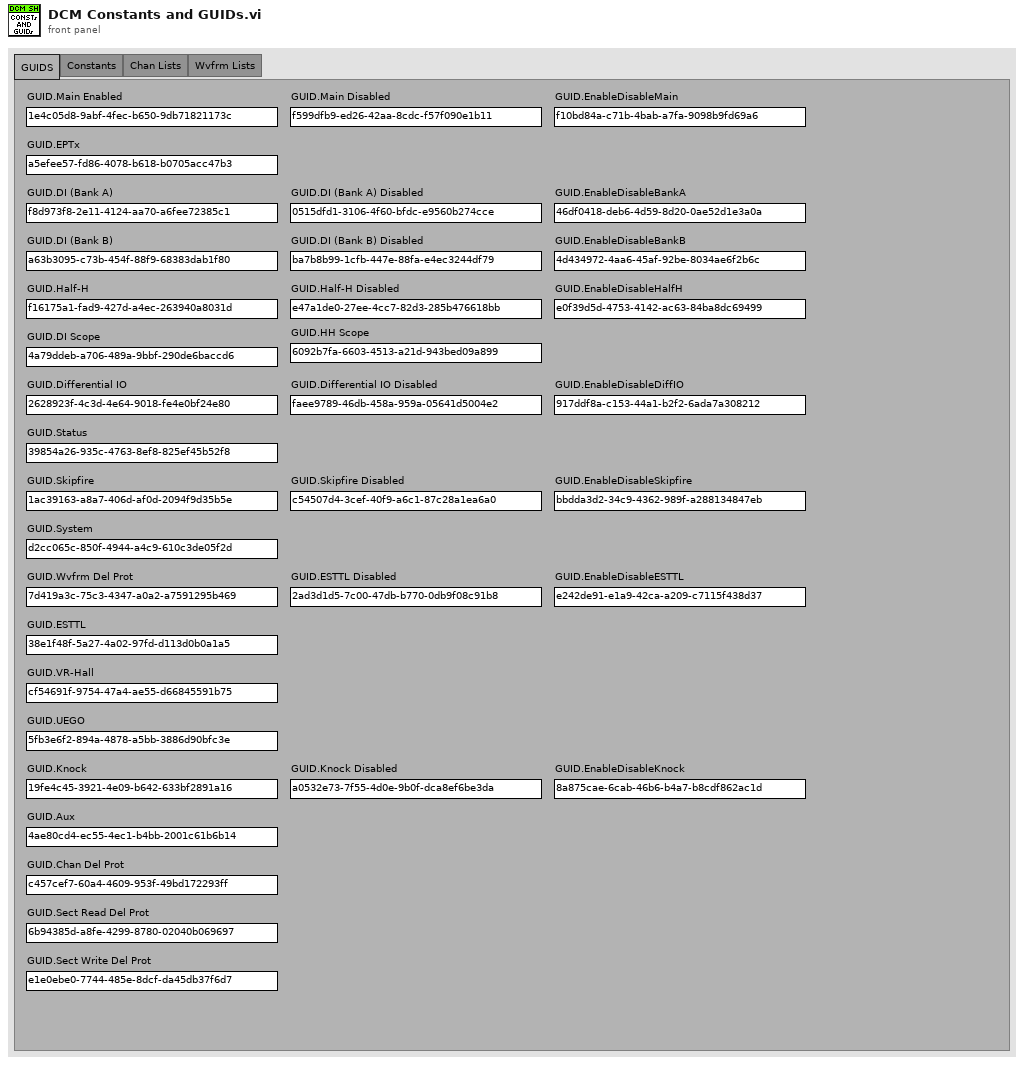
[diagram p1: front panel]
types:
  T1 = enum32{"GUIDS", "Constants", "Chan Lists", "Wvfrm Lists"}
  T2 = typedef "DCM Shared.lvlib/Channel.ctl" = cluster{"Name":string, "Units":string, "Default":dbl, "Description":string}
diagram:
